vi "Find Repeating Length from Direction.vi"(6 "Tolerance":dbl=0.1, 8 "Lattice vector c":dbl[](array[numeric])=[0.0, 0.0, 6.615785553057252], 9 "Lattice vector b":dbl[](array[numeric])=[0.0, 6.615785553057252, 0.0], 10 "Lattice vector a":dbl[](array[numeric])=[6.615785553057252, 0.0, 0.0], 11 "Direction":dbl[](array[numeric])=[1.0, 0.0, 0.0]) -> (3 "Repeating Length (A)":dbl=6.615785553057252)   [LabVIEW 2010]
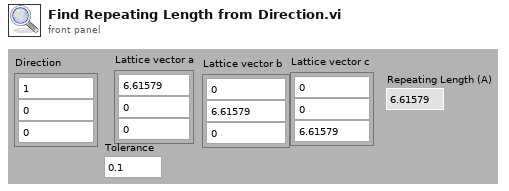
[diagram p1: front panel]
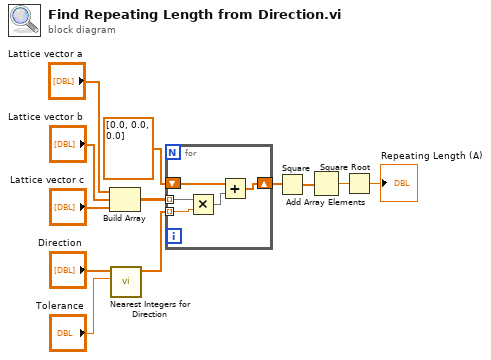
[diagram p0: block diagram]
diagram:
  n1 = Build Array("Lattice vector a", "Lattice vector b", "Lattice vector c") -> (w12:dbl[][])
  n2 = call "Nearest Integers for Direction.vi"("Tolerance"="Tolerance", "Direction"="Direction") -> ("Nearest Integer Directions"=w1:dbl[])  [unwired: 8 in, 1 out]
  n3 = for {
    tunnel: w1 -> [w17] mode=indexing
    tunnel: w12 -> [w16] mode=indexing
    shift-right: [w14] -> w10
    shift-left: dbl[] [0.0, 0.0, 0.0] -> [w13]
    n4 = Multiply(x=w16, y=w17) -> (x*y=w15:dbl[])
    n5 = Add(x=w13, y=w15) -> (x+y=w14:dbl[])
  }
  n6 = Square(x=w10) -> (x^2=w9:dbl[])
  n7 = Add Array Elements(numeric array=w9) -> (sum=w8:dbl)
  n8 = Square Root(x=w8) -> (sqrt(x)=→"Repeating Length (A)":dbl)
